vi "Excute.vi"(8 "error in (no error)":errorcluster, 11 "BeforeDecorator in":refnum<class "BeforeDecorator.lvclass">) -> (0 "error out":errorcluster, 3 "BeforeDecorator out":refnum<class "BeforeDecorator.lvclass">)   [LabVIEW 2014, in "BeforeDecorator.lvclass"]
uses:
  BeforeDecorator.lvclass
  Decorator_class/Decorator.lvclass
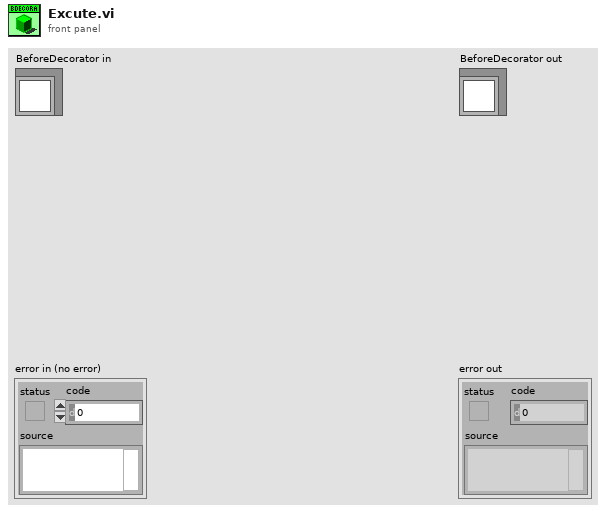
[diagram p1: front panel]
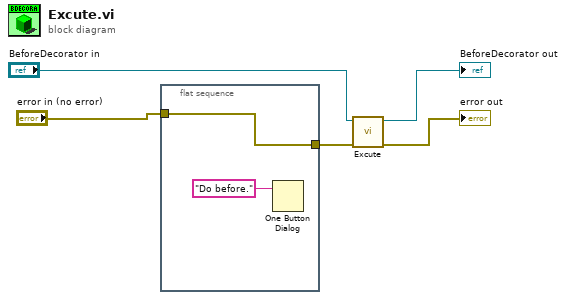
[diagram p0: block diagram]
diagram:
  n1 = flat-sequence {
    tunnel: [w6] -> w2
    tunnel: "error in (no error)" -> [w6]
    frame #0 {
      n2 = One Button Dialog(message="Do before.") -> ()  [unwired: 1 in, 1 out]
    }
  }
  n3 = call-parent "Excute.vi"("error in (no error)"=w2, "Decorator in"="BeforeDecorator in") -> ("error out"=→"error out":errorcluster, "Decorator out"=→"BeforeDecorator out":refnum<class "BeforeDecorator.lvclass">)  [unwired: 8 in]
